vi "Trajectory_Concatenate.vi"(9 "InputTRAJECTORY 2":T1 {"States"."POSE"."ROTATION"."SIN" format="%13.4f"; "States"."POSE"."ROTATION"."COS" format="%13.4f"; "States"."POSE"."ROTATION"."VALUE" format="%13.4f"; "States"."POSE"."TRANSLATION"."Y" format="%14.3f"; "States"."POSE"."TRANSLATION"."X" format="%14.3f"; "TotalTImeSecs" format="%20.3f"}, 11 "InputTRAJECTORY":T1 {"States"."POSE"."ROTATION"."SIN" format="%13.4f"; "States"."POSE"."ROTATION"."COS" format="%13.4f"; "States"."POSE"."ROTATION"."VALUE" format="%13.4f"; "States"."POSE"."TRANSLATION"."Y" format="%14.3f"; "States"."POSE"."TRANSLATION"."X" format="%14.3f"; "TotalTImeSecs" format="%20.3f"}) -> (3 "outputTRAJECTORY":T1 {"States"."POSE"."ROTATION"."SIN" format="%13.4f"; "States"."POSE"."ROTATION"."COS" format="%13.4f"; "States"."POSE"."ROTATION"."VALUE" format="%13.4f"; "States"."POSE"."TRANSLATION"."Y" format="%14.3f"; "States"."POSE"."TRANSLATION"."X" format="%14.3f"; "TotalTImeSecs" format="%20.3f"})   [LabVIEW 2019, in "Trajectory_Library.lvlib"]
doc: "Concatenates another trajectory to the current trajectory. The user is responsible for making sure that the end pose of this trajectory and the start pose of the other trajectory match (if that is the desired behavior).\n \nInputs:\n - Trajectory 1 -- Initial trajectory\n - Trajectory 2 -- Trajectory to add to end of Trajectory 1\n\nOutputs:\n - OutTrajectory -- Concatenated trajectory"
uses:
  TRAJECTORY.ctl
  TRAJ_STATE.ctl
  POSE2D.ctl
  TRANSLATION2D.ctl
  ROTATION2D.ctl
  Trajectory_Library.lvlib
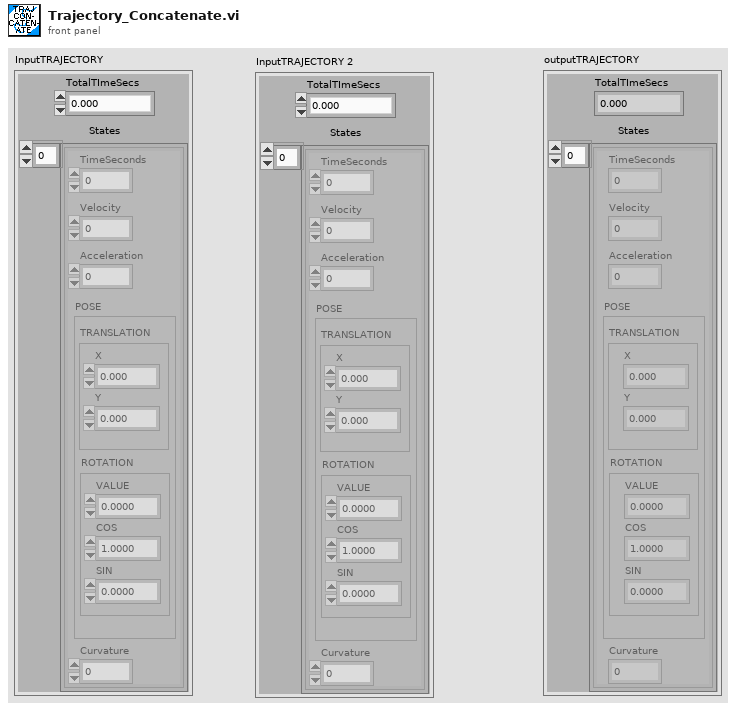
[diagram p1: front panel]
types:
  T1 = typedef "Trajectory_Library.lvlib/TRAJECTORY.ctl" = cluster{"TotalTImeSecs":dbl, "States":T2[]}
  T2 = typedef "Trajectory_Library.lvlib/TRAJ_STATE.ctl" = cluster{"TimeSeconds":dbl, "Velocity":dbl, "Acceleration":dbl, "POSE":T3, "Curvature":dbl}
  T3 = typedef "Trajectory_Library.lvlib/POSE2D.ctl" = cluster{"TRANSLATION":T4, "ROTATION":T5}
  T4 = typedef "Trajectory_Library.lvlib/TRANSLATION2D.ctl" = cluster{"X":dbl, "Y":dbl}
  T5 = typedef "Trajectory_Library.lvlib/ROTATION2D.ctl" = cluster{"VALUE":dbl, "COS":dbl, "SIN":dbl}
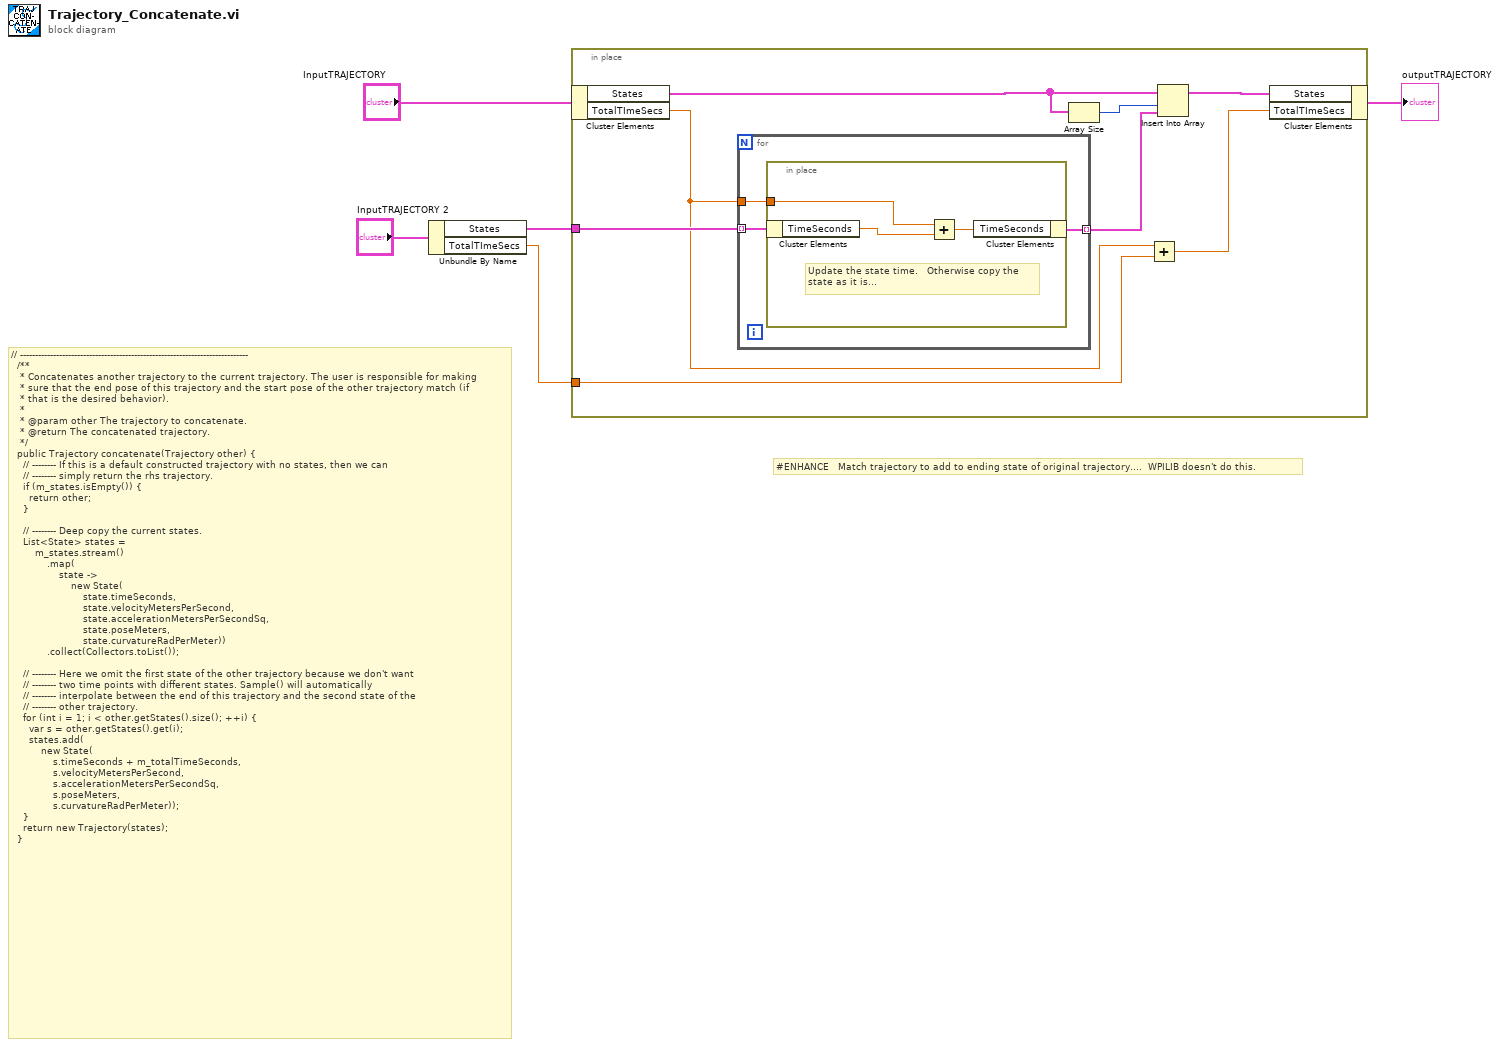
[diagram p0: block diagram]
diagram:
  # "#ENHANCE   Match trajectory to add to ending state of original trajectory....  WPILIB doesn't do this."
  # "// ----------------------------------------------------------------------------\n  /**\n   * Concatenates another trajectory to the current trajectory. The user is responsible for making\n   * sure that the end pose of this trajectory and the start pose of the other trajectory match (if\n   * that is the desired behavior).\n   *\n   * @param other The trajectory to concatenate.\n   * @return The concatenated trajectory.\n   */\n  public Trajectory concatenate(Trajectory other) {\n    // -------- If this is a default constructed trajectory with no states, then we can\n    // -------- simply return the rhs trajectory.\n    if (m_states.isEmpty()) {\n      return other;\n    }\n\n    // -------- Deep copy the current states.\n    List<State> states =\n        m_states.stream()\n            .map(\n                state ->\n                    new State(\n                        state.timeSeconds,\n                        state.velocityMetersPerSecond,\n                        state.accelerationMetersPerSecondSq,\n                        state.poseMeters,\n                        state.curvatureRadPerMeter))\n            .collect(Collectors.toList());\n\n    // -------- Here we omit the first state of the other trajectory because we don't want\n    // -------- two time points with different states. Sample() will automatically\n    // -------- interpolate between the end of this trajectory and the second state of the\n    // -------- other trajectory.\n    for (int i = 1; i < other.getStates().size(); ++i) {\n      var s = other.getStates().get(i);\n      states.add(\n          new State(\n              s.timeSeconds + m_totalTimeSeconds,\n              s.velocityMetersPerSecond,\n              s.accelerationMetersPerSecondSq,\n              s.poseMeters,\n              s.curvatureRadPerMeter));\n    }\n    return new Trajectory(states);\n  }"
  n1 = Unbundle By Name("InputTRAJECTORY 2") -> ("States"=w2:T2[], "TotalTImeSecs"=w1:dbl)
  n2 = in-place {
    in-place-border: w2 -> [w13]
    in-place-border: w1 -> [w10]
    n3 = in-place-cluster #1("InputTRAJECTORY") -> ("States"=w7:T2[], "TotalTImeSecs"=w9:dbl)
    n4 = for {
      tunnel: w13 -> [w16] mode=indexing
      tunnel: w9 -> [w15]
      tunnel: [w14] -> w12 mode=indexing
      n5 = in-place {
        in-place-border: w15 -> [w18]
        # "Update the state time.   Otherwise copy the \nstate as it is..."
        n6 = in-place-cluster #2(w16) -> ("TimeSeconds"=w17:dbl)
        n7 = Add(x=w18, y=w17) -> (x+y=w19:dbl)
        n8 = in-place-cluster #2("TimeSeconds"=w19) -> (w14:T2)
      }
    }
    n9 = Array Size(array=w7) -> (size(s)=w6:i32)
    n10 = Add(x=w9, y=w10) -> (x+y=w8:dbl)
    n11 = Insert Into Array(array=w7, index=w6, new element=w12) -> (w11:T2[])
    n12 = in-place-cluster #1("States"=w11, "TotalTImeSecs"=w8) -> (→"outputTRAJECTORY":T1)
  }
